vi "Graph_Water_Velocity(Subvi).vi"(0 "ItemNames 2":string[][](array[string]), 5 "ItemNames":string[][](array[string])) -> (1 "Water_Velocity":dbl, 3 "Water_Velocity 2":dbl, 4 "Water_Velocity 10":dbl, 6 "Water_Velocity 3":dbl, 8 "Water_Velocity 9":dbl, 10 "Water_Velocity 4":dbl, 12 "Water_Velocity 8":dbl, 13 "Water_Velocity 7":dbl, 14 "Water_Velocity 6":dbl, 15 "Water_Velocity 5":dbl)   [LabVIEW 2024]
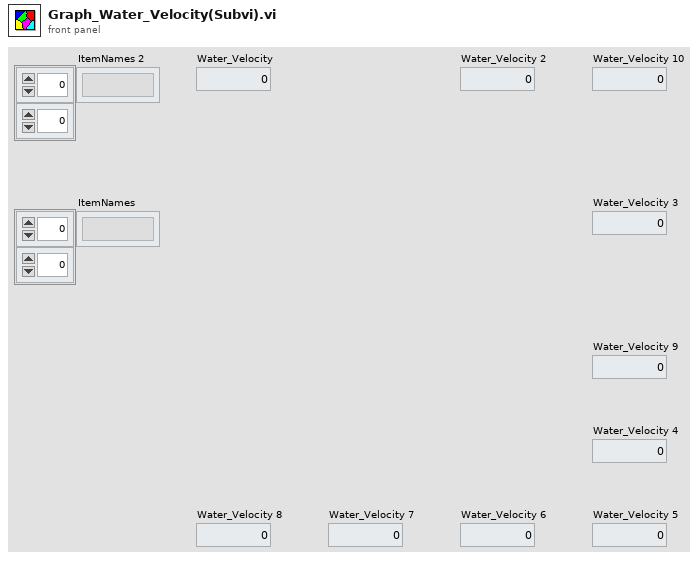
[diagram p1: front panel]
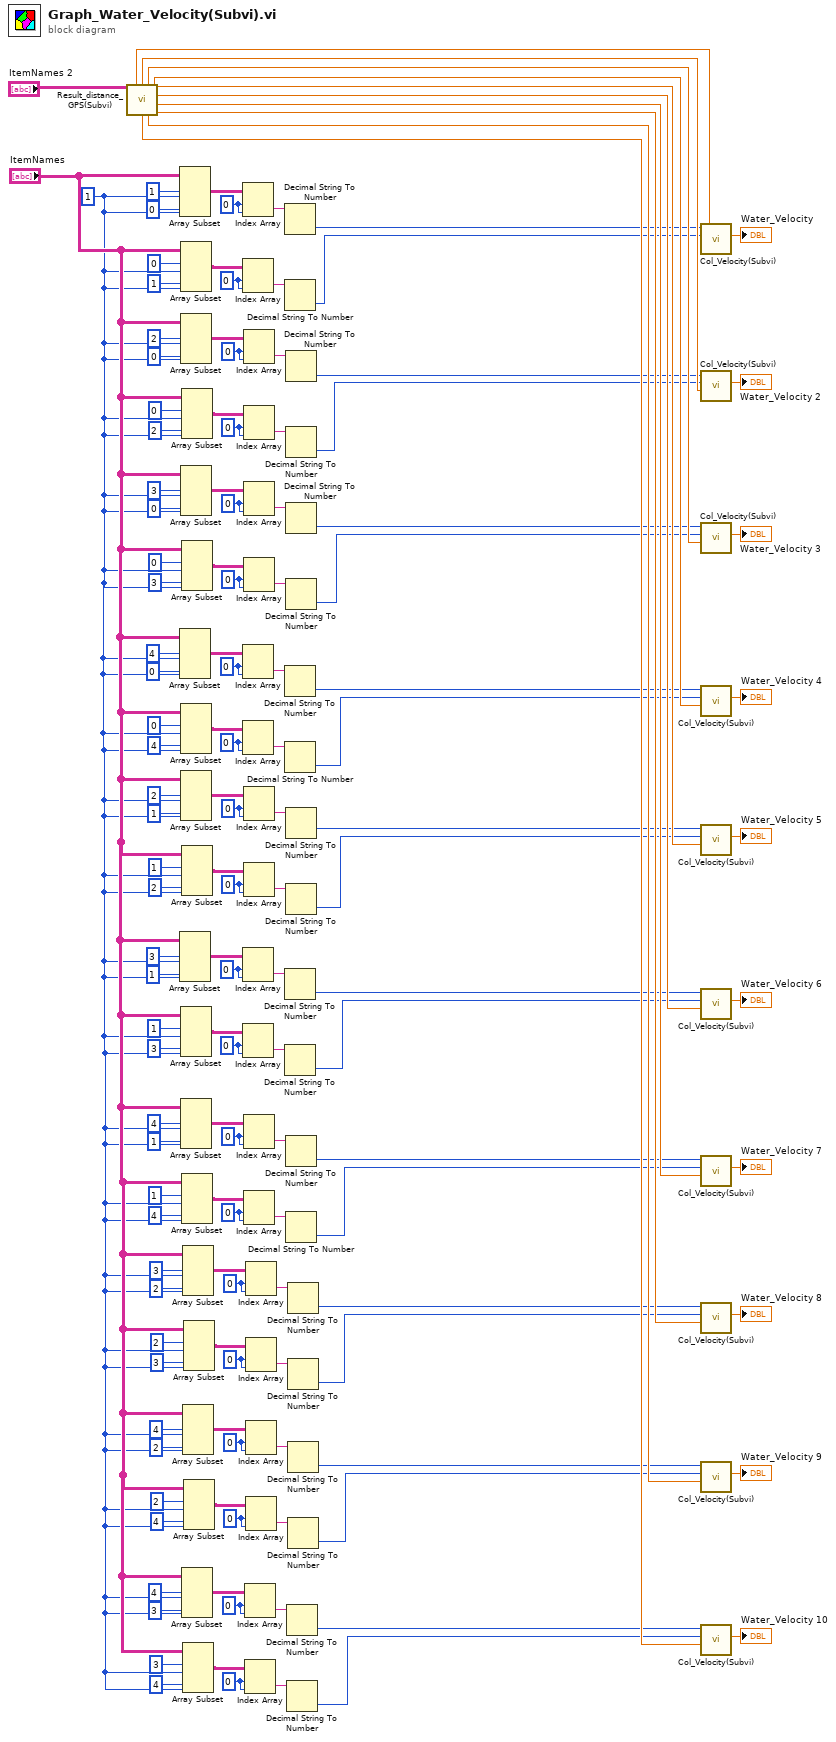
[diagram p0: block diagram]
diagram:
  w120 = 0 ("인덱스 (행)")
  w123 = 0 ("인덱스 (행)")
  w114 = 0 ("인덱스 (행)")
  w111 = 0 ("인덱스 (행)")
  w94 = 0 ("인덱스 (행)")
  w97 = 0 ("인덱스 (행)")
  w88 = 0 ("인덱스 (행)")
  w85 = 0 ("인덱스 (행)")
  w68 = 0 ("인덱스 (행)")
  w71 = 0 ("인덱스 (행)")
  w62 = 0 ("인덱스 (행)")
  w59 = 0 ("인덱스 (행)")
  w42 = 0 ("인덱스 (행)")
  w45 = 0 ("인덱스 (행)")
  w36 = 0 ("인덱스 (행)")
  w33 = 0 ("인덱스 (행)")
  w16 = 0 ("인덱스 (행)")
  w19 = 0 ("인덱스 (행)")
  w10 = 0 ("인덱스 (행)")
  w7 = 0 ("인덱스 (행)")
  w129 = 1 ("길이")
  n1 = call "Result_distance_GPS(Subvi).vi"("아이템 이름"="ItemNames 2") -> ("1_2_distance[m]"=w14:dbl, "1_3_distance[m]"=w27:dbl, "1_4_distance[m]"=w40:dbl, "1_5_distance[m]"=w53:dbl, "2_3_distance[m]"=w66:dbl, "2_4_distance[m]"=w79:dbl, "2_5_distance[m]"=w92:dbl, "4_5_distance[m]"=w132:dbl, "3_5_distance[m]"=w118:dbl, "3_4_distance[m]"=w105:dbl)  [unwired: 5 in]
  n2 = Array Subset(array="ItemNames", index (row)=1 ("인덱스"), length (row)=w129, index (col)=0 ("인덱스"), length (col)=w129) -> (w6:string[][])
  n3 = Array Subset(array="ItemNames", index (row)=4 ("인덱스"), length (row)=w129, index (col)=0 ("인덱스"), length (col)=w129) -> (w46:string[][])
  n4 = Array Subset(array="ItemNames", index (row)=3 ("인덱스"), length (row)=w129, index (col)=1 ("인덱스"), length (col)=w129) -> (w72:string[][])
  n5 = Array Subset(array="ItemNames", index (row)=0 ("인덱스"), length (row)=w129, index (col)=1 ("인덱스"), length (col)=w129) -> (w11:string[][])
  n6 = Array Subset(array="ItemNames", index (row)=2 ("인덱스"), length (row)=w129, index (col)=0 ("인덱스"), length (col)=w129) -> (w20:string[][])
  n7 = Array Subset(array="ItemNames", index (row)=3 ("인덱스"), length (row)=w129, index (col)=0 ("인덱스"), length (col)=w129) -> (w32:string[][])
  n8 = Array Subset(array="ItemNames", index (row)=0 ("인덱스"), length (row)=w129, index (col)=4 ("인덱스"), length (col)=w129) -> (w41:string[][])
  n9 = Array Subset(array="ItemNames", index (row)=2 ("인덱스"), length (row)=w129, index (col)=1 ("인덱스"), length (col)=w129) -> (w58:string[][])
  n10 = Array Subset(array="ItemNames", index (row)=1 ("인덱스"), length (row)=w129, index (col)=3 ("인덱스"), length (col)=w129) -> (w67:string[][])
  n11 = Array Subset(array="ItemNames", index (row)=4 ("인덱스"), length (row)=w129, index (col)=1 ("인덱스"), length (col)=w129) -> (w84:string[][])
  n12 = Array Subset(array="ItemNames", index (row)=0 ("인덱스"), length (row)=w129, index (col)=2 ("인덱스"), length (col)=w129) -> (w15:string[][])
  n13 = Array Subset(array="ItemNames", index (row)=0 ("인덱스"), length (row)=w129, index (col)=3 ("인덱스"), length (col)=w129) -> (w37:string[][])
  n14 = Array Subset(array="ItemNames", index (row)=1 ("인덱스"), length (row)=w129, index (col)=2 ("인덱스"), length (col)=w129) -> (w63:string[][])
  n15 = Array Subset(array="ItemNames", index (row)=1 ("인덱스"), length (row)=w129, index (col)=4 ("인덱스"), length (col)=w129) -> (w89:string[][])
  n16 = Array Subset(array="ItemNames", index (row)=4 ("인덱스"), length (row)=w129, index (col)=3 ("인덱스"), length (col)=w129) -> (w124:string[][])
  n17 = Array Subset(array="ItemNames", index (row)=3 ("인덱스"), length (row)=w129, index (col)=2 ("인덱스"), length (col)=w129) -> (w98:string[][])
  n18 = Array Subset(array="ItemNames", index (row)=4 ("인덱스"), length (row)=w129, index (col)=2 ("인덱스"), length (col)=w129) -> (w110:string[][])
  n19 = Array Subset(array="ItemNames", index (row)=3 ("인덱스"), length (row)=w129, index (col)=4 ("인덱스"), length (col)=w129) -> (w119:string[][])
  n20 = Array Subset(array="ItemNames", index (row)=2 ("인덱스"), length (row)=w129, index (col)=3 ("인덱스"), length (col)=w129) -> (w93:string[][])
  n21 = Array Subset(array="ItemNames", index (row)=2 ("인덱스"), length (row)=w129, index (col)=4 ("인덱스"), length (col)=w129) -> (w115:string[][])
  n22 = Index Array(array=w6, index (row)=w7, index (col)=w7) -> (element=w8:string)
  n23 = Index Array(array=w11, index (row)=w10, index (col)=w10) -> (element=w9:string)
  n24 = Index Array(array=w46, index (row)=w45, index (col)=w45) -> (element=w44:string)
  n25 = Index Array(array=w41, index (row)=w42, index (col)=w42) -> (element=w43:string)
  n26 = Index Array(array=w72, index (row)=w71, index (col)=w71) -> (element=w70:string)
  n27 = Index Array(array=w67, index (row)=w68, index (col)=w68) -> (element=w69:string)
  n28 = Index Array(array=w20, index (row)=w19, index (col)=w19) -> (element=w18:string)
  n29 = Index Array(array=w15, index (row)=w16, index (col)=w16) -> (element=w17:string)
  n30 = Index Array(array=w32, index (row)=w33, index (col)=w33) -> (element=w34:string)
  n31 = Index Array(array=w37, index (row)=w36, index (col)=w36) -> (element=w35:string)
  n32 = Index Array(array=w58, index (row)=w59, index (col)=w59) -> (element=w60:string)
  n33 = Index Array(array=w63, index (row)=w62, index (col)=w62) -> (element=w61:string)
  n34 = Index Array(array=w84, index (row)=w85, index (col)=w85) -> (element=w86:string)
  n35 = Index Array(array=w89, index (row)=w88, index (col)=w88) -> (element=w87:string)
  n36 = Index Array(array=w124, index (row)=w123, index (col)=w123) -> (element=w122:string)
  n37 = Index Array(array=w119, index (row)=w120, index (col)=w120) -> (element=w121:string)
  n38 = Index Array(array=w98, index (row)=w97, index (col)=w97) -> (element=w96:string)
  n39 = Index Array(array=w93, index (row)=w94, index (col)=w94) -> (element=w95:string)
  n40 = Index Array(array=w110, index (row)=w111, index (col)=w111) -> (element=w112:string)
  n41 = Index Array(array=w115, index (row)=w114, index (col)=w114) -> (element=w113:string)
  n42 = Decimal String To Number(string=w8) -> (number=w12:i32)  [unwired: 2 in, 1 out]
  n43 = Decimal String To Number(string=w9) -> (number=w13:i32)  [unwired: 2 in, 1 out]
  n44 = Decimal String To Number(string=w44) -> (number=w51:i32)  [unwired: 2 in, 1 out]
  n45 = Decimal String To Number(string=w43) -> (number=w52:i32)  [unwired: 2 in, 1 out]
  n46 = Decimal String To Number(string=w70) -> (number=w77:i32)  [unwired: 2 in, 1 out]
  n47 = Decimal String To Number(string=w69) -> (number=w78:i32)  [unwired: 2 in, 1 out]
  n48 = Decimal String To Number(string=w18) -> (number=w25:i32)  [unwired: 2 in, 1 out]
  n49 = Decimal String To Number(string=w17) -> (number=w26:i32)  [unwired: 2 in, 1 out]
  n50 = Decimal String To Number(string=w34) -> (number=w38:i32)  [unwired: 2 in, 1 out]
  n51 = Decimal String To Number(string=w35) -> (number=w39:i32)  [unwired: 2 in, 1 out]
  n52 = Decimal String To Number(string=w60) -> (number=w64:i32)  [unwired: 2 in, 1 out]
  n53 = Decimal String To Number(string=w61) -> (number=w65:i32)  [unwired: 2 in, 1 out]
  n54 = Decimal String To Number(string=w86) -> (number=w90:i32)  [unwired: 2 in, 1 out]
  n55 = Decimal String To Number(string=w87) -> (number=w91:i32)  [unwired: 2 in, 1 out]
  n56 = Decimal String To Number(string=w122) -> (number=w130:i32)  [unwired: 2 in, 1 out]
  n57 = Decimal String To Number(string=w121) -> (number=w131:i32)  [unwired: 2 in, 1 out]
  n58 = Decimal String To Number(string=w96) -> (number=w103:i32)  [unwired: 2 in, 1 out]
  n59 = Decimal String To Number(string=w95) -> (number=w104:i32)  [unwired: 2 in, 1 out]
  n60 = Decimal String To Number(string=w112) -> (number=w116:i32)  [unwired: 2 in, 1 out]
  n61 = Decimal String To Number(string=w113) -> (number=w117:i32)  [unwired: 2 in, 1 out]
  n62 = call "Col_Velocity(Subvi).vi"("거리"=w14, "Station_index_2"=w13, "Station_index_1"=w12) -> ("Water_Velocity"=→"Water_Velocity":dbl)  [unwired: 7 in, 1 out]
  n63 = call "Col_Velocity(Subvi).vi"("거리"=w27, "Station_index_2"=w26, "Station_index_1"=w25) -> ("Water_Velocity"=→"Water_Velocity 2":dbl)  [unwired: 7 in, 1 out]
  n64 = call "Col_Velocity(Subvi).vi"("거리"=w40, "Station_index_2"=w39, "Station_index_1"=w38) -> ("Water_Velocity"=→"Water_Velocity 3":dbl)  [unwired: 7 in, 1 out]
  n65 = call "Col_Velocity(Subvi).vi"("거리"=w53, "Station_index_2"=w52, "Station_index_1"=w51) -> ("Water_Velocity"=→"Water_Velocity 4":dbl)  [unwired: 7 in, 1 out]
  n66 = call "Col_Velocity(Subvi).vi"("거리"=w66, "Station_index_2"=w65, "Station_index_1"=w64) -> ("Water_Velocity"=→"Water_Velocity 5":dbl)  [unwired: 7 in, 1 out]
  n67 = call "Col_Velocity(Subvi).vi"("거리"=w79, "Station_index_2"=w78, "Station_index_1"=w77) -> ("Water_Velocity"=→"Water_Velocity 6":dbl)  [unwired: 7 in, 1 out]
  n68 = call "Col_Velocity(Subvi).vi"("거리"=w92, "Station_index_2"=w91, "Station_index_1"=w90) -> ("Water_Velocity"=→"Water_Velocity 7":dbl)  [unwired: 7 in, 1 out]
  n69 = call "Col_Velocity(Subvi).vi"("거리"=w105, "Station_index_2"=w104, "Station_index_1"=w103) -> ("Water_Velocity"=→"Water_Velocity 8":dbl)  [unwired: 7 in, 1 out]
  n70 = call "Col_Velocity(Subvi).vi"("거리"=w118, "Station_index_2"=w117, "Station_index_1"=w116) -> ("Water_Velocity"=→"Water_Velocity 9":dbl)  [unwired: 7 in, 1 out]
  n71 = call "Col_Velocity(Subvi).vi"("거리"=w132, "Station_index_2"=w131, "Station_index_1"=w130) -> ("Water_Velocity"=→"Water_Velocity 10":dbl)  [unwired: 7 in, 1 out]
